vi "INI Initialize Extensions Global.vi"(11 "Error In (no error)":errorcluster) -> (15 "Error Out":errorcluster)   [LabVIEW 2011]
doc: "This routine is used to initialize the ini file portion of the system which handles pre-defined types, and enumerated types in the controls registry."
uses:
  File IO/Type Defs/FILE Type Enum.ctl
  INI Extensions Global.vi
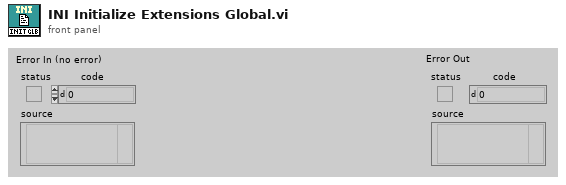
[diagram p1: front panel]
types:
  T1 = typedef "INI Extensions Cluster.ctl" = cluster{"Type Descriptions Path":path, "Pre-Defined Type Names":string[], "Pre-Defined Type Info":string[], "Text Lists":string[]}
  T2 = typedef "FILE Type Enum.ctl" = enum16{"Text", "Spreadsheet"}
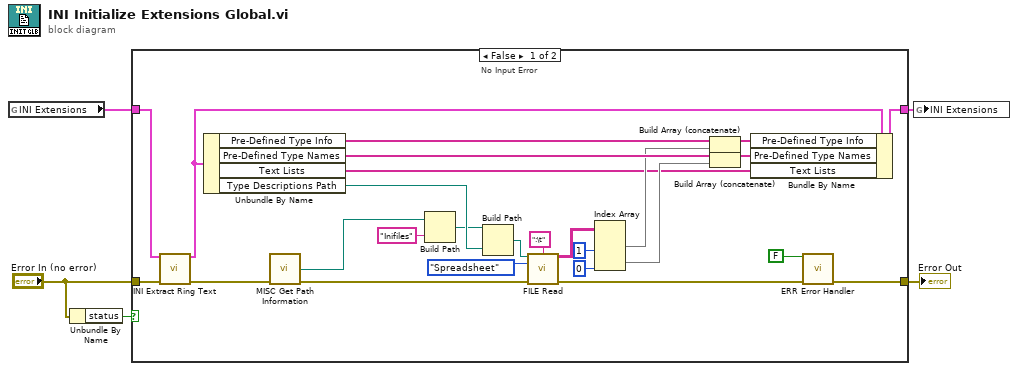
[diagram p0: block diagram]
diagram:
  n1 = global read "INI Extensions Global.vi" "INI Extensions"() -> (w2:T1)
  n2 = Unbundle By Name("Error In (no error)") -> ("status"=w5:bool)
  n3 = case shown="False" w5 {
    tunnel: [w27 w33] -> w4
    tunnel: "Error In (no error)" -> [w30 w33]
    tunnel: w2 -> [w31 w32]
    tunnel: [w28 w32] -> w1
    frame False {
      # "No Input Error"
      n4 = call "INI Extract Ring Text.vi"("INI Extensions In"=w31, "Error In (no error)"=w30) -> ("INI Extensions Out"=w29:T1, "Error Out"=w10:errorcluster)  [unwired: 12 out]
      n5 = Unbundle By Name(w29) -> ("Pre-Defined Type Info"=w20:string[], "Pre-Defined Type Names"=w19:string[], "Text Lists"=w11:string[], "Type Descriptions Path"=w25:path)
      n6 = call "MISC Get Path Information.vi"("Error In (no error)"=w10) -> ("Support Directory"=w8:path, "Error Out"=w9:errorcluster)  [unwired: 13 out]
      n7 = Build Path(base path=w8, name or relative path="Inifiles") -> (appended path=w6:path)
      n8 = Build Path(base path=w6, name or relative path=w25) -> (appended path=w24:path)
      n9 = call "FILE Read.vi"("File Path (dialog if empty)"=w24, "Delimiter (Tab)"=":\t", "File Type (text)"=FILE_Type_Enum."Spreadsheet", "Error In (no error)"=w9) -> ("Spreadsheet Data (all)"=w16:string[][], "Error Out"=w21:errorcluster)  [unwired: 3 in, 7 out]
      n10 = Index Array(array=w16, index (col) #1=1 ("disabled index (col)"), index (col) #2=0 ("index (col)")) -> (element #1=w13:string[], element #2=w12:string[])  [unwired: 2 in]
      n11 = Build Array (concatenate)(w20, w13) -> (w23:string[])
      n12 = Build Array (concatenate)(w19, w12) -> (w22:string[])
      n13 = Bundle By Name(cluster=w29, "Pre-Defined Type Info"=w23, "Pre-Defined Type Names"=w22, "Text Lists"=w11) -> (w28:T1)
      n14 = call "ERR Error Handler.vi"("Error Status"=FALSE ("Error Flag"), "Error In (no error)"=w21) -> ("Error Out"=w27:errorcluster)  [unwired: 4 in, 9 out]
    }
    frame True {
      # "Input Error"
    }
  }
  "Error Out" <- w4
  n15 = global write "INI Extensions Global.vi" "INI Extensions"(w1) -> ()
